vi "YPR range coerce.vi"(8 "Error In":errorcluster, 10 "YPR data":cluster{"Yaw":sgl, "Pitch":sgl, "Roll":sgl}) -> (0 "Error Out":errorcluster, 2 "YPR Array":sgl[](array[numeric]))   [LabVIEW 2016]
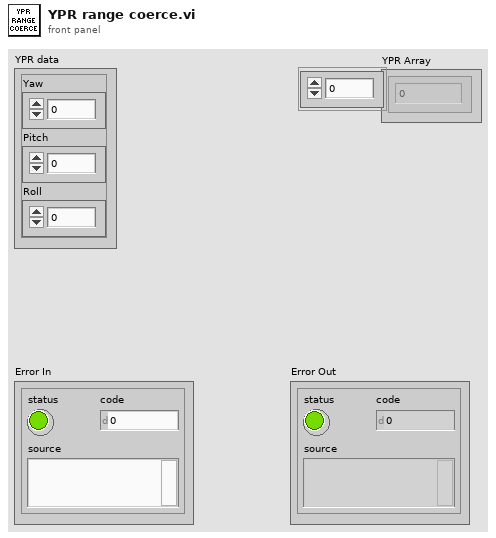
[diagram p1: front panel]
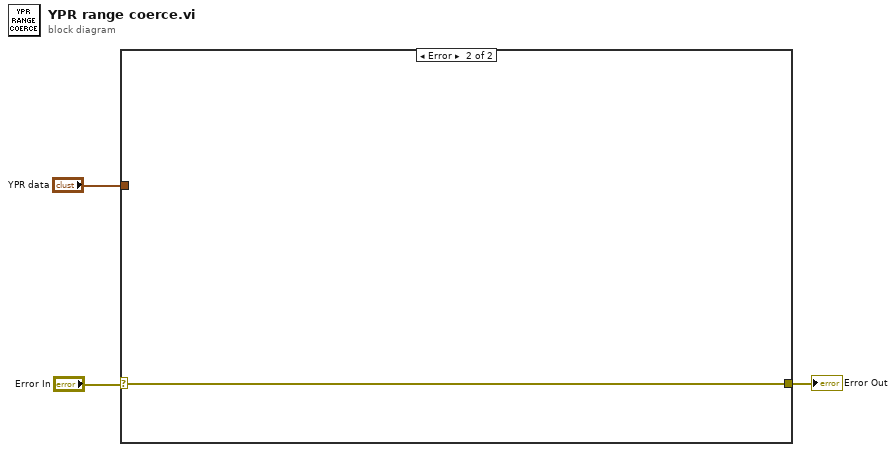
[diagram p0: block diagram]
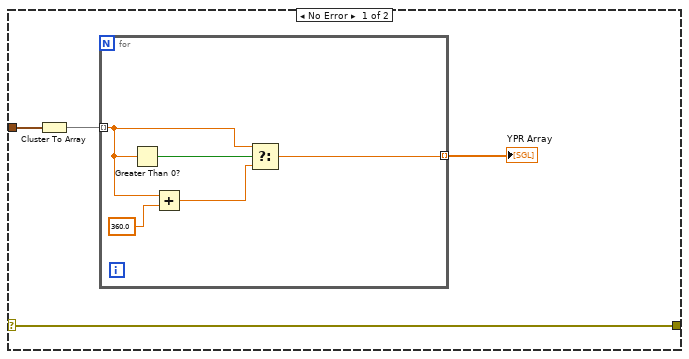
[diagram p2: hidden frame]
diagram:
  n1 = case shown="Error" "Error In" {
    selector: "Error In" -> [w7 w13]
    tunnel: [w7 w13] -> w2
    tunnel: "YPR data" -> [w6 _]
    frame No Error {
      n2 = Cluster To Array(cluster=w6) -> (array=w5:sgl[])
      n3 = for {
        tunnel: w5 -> [w11] mode=indexing
        tunnel: [w8] -> w4 mode=indexing
        n4 = Greater Than 0?(x=w11) -> (x > 0?=w12:bool)
        n5 = Add(x=w11, y=sgl 360.0) -> (x+y=w9:sgl)
        n6 = Select(t=w11, s=w12, f=w9) -> (s? t:f=w8:sgl)
      }
      "YPR Array" <- w4
    }
    frame Error {
    }
  }
  "Error Out" <- w2
